vi "ReadEncoders.vi"(8 "error in (no error)":errorcluster, 11 "Pod Drive in":refnum<class "Pod Drive.lvclass">) -> (0 "error out":errorcluster, 1 "Right Encoder":i32, 2 "Left Encoder":i32, 3 "Pod Drive out":refnum<class "Pod Drive.lvclass">)   [LabVIEW 2018, in "Drive.lvlib" / "Pod Drive.lvclass"]
doc: "Reads the encoders on the drive talons and gets their encoder ticks in talon native units"
uses:
  Pod Drive.lvclass
  Pod Drive.lvclass/Pod Drive.ctl
  <vilib>/Rock Robotics/WPI/ThirdParty/Phoenix-LabVIEW/Motor Controller/Get/CTRE_Phoenix_MotorController_GetSelectedSensorData.vi
  Drive.lvclass
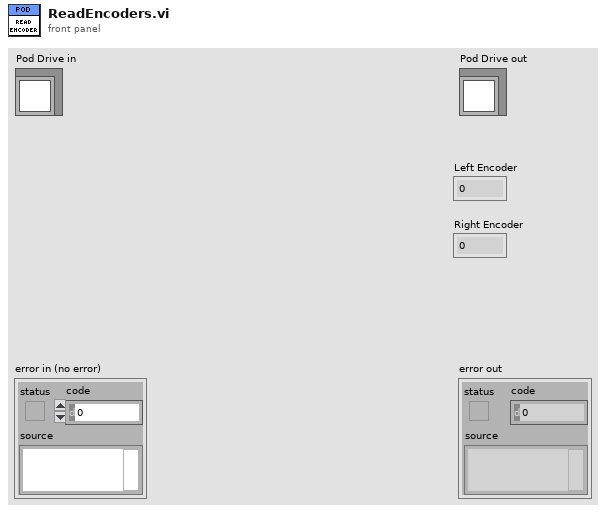
[diagram p1: front panel]
types:
  T1 = typedef "WPI_MotorControlDeviceRef.ctl" = cluster{"DeviceStatus":errorcluster, "Type":T2, "PWM":cluster{"PWM Channel":T3, "DeadBand":T4}, "CAN":cluster{"Device Number":u8, "SetOutput VI Ref":variant, "GetOutput VI Ref":variant, "Enable VI Ref":variant, "Disable VI Ref":variant, "Data":variant}, "Invert":bool, "DIO PWM":cluster{"PWM \"Enable\" Channel":T3, "DIOChannel":T5, "PWM Rate":dbl}}
  T2 = typedef "WPI_MotorControlType.ctl" = enum16{"PWM", "CAN", "DIO PWM"}
  T3 = typedef "FPGA_DIOPWMChannel.ctl" = enum8{"PWM 0", "PWM 1", "PWM 2", "PWM 3", "PWM 4", "PWM 5", "PWM 6", "PWM 7", "PWM 8", "PWM 9", "PWM MXP 0", "PWM MXP 1", "PWM MXP 2", "PWM MXP 3", "PWM MXP 4", "PWM MXP 5", "PWM MXP 6", "PWM MXP 7", "PWM MXP 8", "PWM MXP 9", "Invalid"}
  T4 = typedef "WPI_PWMDeadband.ctl" = cluster{"Name":string, "maxPositivePwm":i32, "minPositivePwm":i32, "centerPwm":i32, "maxNegativePwm":i32, "minNegativePwm":i32, "angularRange":u16}
  T5 = typedef "FPGA_DIOChannel.ctl" = enum8{"DIO 0", "DIO 1", "DIO 2", "DIO 3", "DIO 4", "DIO 5", "DIO 6", "DIO 7", "DIO 8", "DIO 9", "DIO MXP 0", "DIO MXP 1", "DIO MXP 2", "DIO MXP 3", "DIO MXP 4", "DIO MXP 5", "DIO MXP 6", "DIO MXP 7", "DIO MXP 8", "DIO MXP 9", "DIO MXP 10", "DIO MXP 11", "DIO MXP 12", "DIO MXP 13", "DIO MXP 14", "DIO MXP 15", "SPI Port CS1", "SPI Port CS2", "SPI Port CS3", "SPI Port MISO", "SPI Port MOSI", "Invalid"}
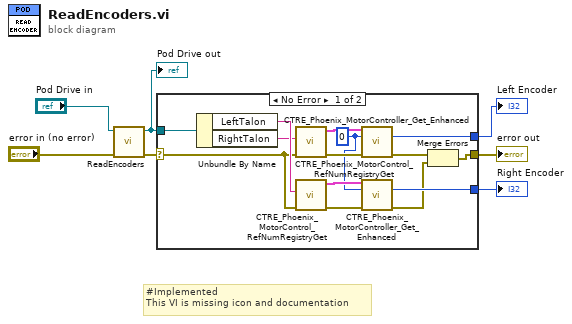
[diagram p0: block diagram]
diagram:
  # "#Implemented\nThis VI is missing icon and documentation"
  n1 = call-parent "ReadEncoders.vi"("error in (no error)"="error in (no error)", "Drive in"="Pod Drive in") -> ("error out"=w5:errorcluster, "Drive out"=w4:refnum<class "Pod Drive.lvclass">)  [unwired: 6 in, 2 out]
  "Pod Drive out" <- w4
  n2 = case shown="No Error" w5 {
    selector: w5 -> [w9 w22]
    tunnel: [w17 _] -> w3
    tunnel: [w16 _] -> w2
    tunnel: [w14 w22] -> w1
    tunnel: w4 -> [w12 _]
    frame No Error {
      w8 = u32 0 ("pidLoopIdx")
      n3 = Unbundle By Name(w12) -> ("LeftTalon"=w11:string, "RightTalon"=w10:string)
      n4 = call <vilib>:"CTRE_Phoenix_MotorControl_RefNumRegistryGet.vi"("error in (no error)"=w9, "refnum name"=w10) -> ("error out"=w20:errorcluster, "PhoenixMotorControlDevRef"=w21:T1)  [unwired: 8 in]
      n5 = call <vilib>:"CTRE_Phoenix_MotorControl_RefNumRegistryGet.vi"("error in (no error)"=w9, "refnum name"=w11) -> ("error out"=w18:errorcluster, "PhoenixMotorControlDevRef"=w19:T1)  [unwired: 8 in]
      n6 = call-poly <vilib>:"CTRE_Phoenix_MotorController_Get_Enhanced.vi"("PhoenixMotorControlDevRef"=w21, "pidLoopIdx"=w8, "error in"=w20) -> ("Position (Raw Sensor Units)"=w17:i32, "error out"=w13:errorcluster)  [unwired: 9 in, 2 out]
      n7 = call-poly <vilib>:"CTRE_Phoenix_MotorController_Get_Enhanced.vi"("PhoenixMotorControlDevRef"=w19, "pidLoopIdx"=w8, "error in"=w18) -> ("Position (Raw Sensor Units)"=w16:i32, "error out"=w15:errorcluster)  [unwired: 9 in, 2 out]
      n8 = Merge Errors(w13, w15) -> (w14:errorcluster)
    }
    frame Error {
    }
  }
  "error out" <- w1
  "Right Encoder" <- w2
  "Left Encoder" <- w3
